vi "basic - VL Transmit.vi"() -> ()   [LabVIEW 2020]
uses:
  src/AIM664LV.lvlib
  src/_polimorphicInstances/session/Fdx Create Session (Tx-UDP Port-Oriented).vi
  src/bsp/AFDX_Transmit/Fdx Create Tx VL.vi
  src/_polimorphicInstances/udpPort/Fdx Create UDP Port (TX-CommPort).vi
  src/_polimorphicInstances/session/Fdx Close Session (Port).vi
  src/_controls/comm_computedMAC-IP.ctl
  src/_controls/comm_udp_tx.ctl
  src/_controls/comm_config_vl_tx.ctl
  src/helpers/EthFrameManagement/controls/mac_src_info_afdx.ctl
  src/helpers/EthFrameManagement/EthFrameManagement.lvlib
panel:
  in  "VlTx (IP Source)":T1={"domainID"=14, "sideID"=2, "locationID"=3, "interfaceID"=0}
  out "Duplicated":bool=TRUE
  in  "VL Configurations":T4(array[cluster])=[{"VL Config"={"VlId"=3, "NumOfSubVl"=2, "rate mS (128)"=128.0, "domainID"=1, "sideID"=1, "locationID"=254, "interfaceID"=1, "NetSelect"=3, "Skew"=0, "MaxFrameLength"=1000, "FrameBufferSize"=0}, "CommPort Config"=[{"PortType"=enum."FDX_UDP_SAMPLING", "partitionID"=0, "SubVlId"=1, "UdpSrcPort"=0, "UdpDstPort"=0, "SampleRateMs"=128.0, "UdpNumBufMessages"=0, "UdpMaxMessageSize"=1000}, {"PortType"=enum."FDX_UDP_SAMPLING", "partitionID"=0, "SubVlId"=2, "UdpSrcPort"=0, "UdpDstPort"=0, "SampleRateMs"=128.0, "UdpNumBufMessages"=0, "UdpMaxMessageSize"=1000}]}, {"VL Config"={"VlId"=70, "NumOfSubVl"=2, "rate mS (128)"=64.0, "domainID"=1, "sideID"=1, "locationID"=1, "interfaceID"=1, "NetSelect"=3, "Skew"=0, "MaxFrameLength"=1000, "FrameBufferSize"=0}, "CommPort Config"=[{"PortType"=enum."FDX_UDP_SAMPLING", "partitionID"=0, "SubVlId"=1, "UdpSrcPort"=0, "UdpDstPort"=0, "SampleRateMs"=128.0, "UdpNumBufMessages"=0, "UdpMaxMessageSize"=1000}, {"PortType"=enum."FDX_UDP_SAMPLING", "partitionID"=0, "SubVlId"=2, "UdpSrcPort"=0, "UdpDstPort"=0, "SampleRateMs"=128.0, "UdpNumBufMessages"=0, "UdpMaxMessageSize"=1000}]}] {"VL Config"."NetSelect" items=["FDX_TX_FRAME_DLY_A"=0, "FDX_TX_FRAME_DLY_B"=1, "FDX_TX_FRAME_BOTH "=3, "FDX_TX_FRAME_ONLY_A"=4, "FDX_TX_FRAME_ONLY_B "=5]; "VL Config"."interfaceID" format="%.0b"}
  in  "millisecond multiple":u32=128
  in  "PortMap":u32
  out "Data size":i32=128
  out "IndexCycleCount":u32[](array[numeric])
  out "MsgCount":u32[](array[numeric])=[13, 13, 21, 21]
  out "CurrentIndex":u32[](array[numeric])
  out "BytesWritten":u32[](array[numeric])=[128, 128, 128, 128]
  in  "Port":u32
  in  "Board":u32
  out "current time":timestamp=timestamp(3763148385.2241025 s since 1904-01-01)
  out "current irig time":T5={"SignOut"=-1509901600, "DayOut"=16, "HourOut"=8, "MinOut"=7, "SecondOut"=53, "MilliSecOut"=368, "MicroSecOut"=508, "NanoSecOut"=600, "InfoOut"=0, "Mode"=3}
  out "CommPort Addresses":T6[](array[typedef])=[{"MACsrc"=[], "IPsrc"="10.14.67.0", "IPdest"="224.224.0.3"}, {"MACsrc"=[], "IPsrc"="10.14.67.0", "IPdest"="224.224.0.3"}, {"MACsrc"=[], "IPsrc"="10.14.67.0", "IPdest"="224.224.0.70"}, {"MACsrc"=[], "IPsrc"="10.14.67.0", "IPdest"="224.224.0.70"}] {"MACsrc" format="%.0x"}
  out "Data":u8[](array[numeric])=[0, 1, 2, 3, 4, 5, 6, 7, 8, 9, 10, 11, 12, 13, 14, 15, 16, 17, 18, 19, 20, 21, 22, 23, 24, 25, 26, 27, 28, 29, 30, 31, 32, 33, 34, 35, 36, 37, 38, 39, 40, 41, 42, 43, 44, 45, 46, 47, 48, 49, 50, 51, 52, 53, 54, 55, 56, 57, 58, 59, 60, 61, 62, 63, 64, 65, 66, 67, 68, 69, 70, 71, 72, 73, 74, 75, 76, 77, 78, 79, 80, 81, 82, 83, 84, 85, 86, 87, 88, 89, 90, 91, 92, 93, 94, 95, 96, 97, 98, 99, 100, 101, 102, 103, 104, 105, 106, 107, 108, 109, 110, 111, 112, 113, 114, 115, 116, 117, 118, 119, 120, 121, 122, 123, 124, 125, 126, 127] format="%.0x"
  in  "stop":bool
  out "PortInitOut":T7={"PortConfig"=0, "PortUsed"=1, "GlobalMemFree"=0, "SharedMemFree"=0} {"PortConfig" items=["FDX_SINGLE", "FDX_REDUNDANT"]}
  out "error out":errorcluster
  # "ARINC 664 - Transmitting through many VL (Virtual Link)"
  # "Overview: Setup the board to transmit package as raw frames.\nRequirement: One AIM ARINC-664 board with installed AIM ARINC 664 BSP.\nRestrictions: None.\nInstruction:\n1. Select the Board ID (0 if you have only one board in your system) and the port number. If you want to validate between two ports in one device, you can use tx board and Rx Board\n2. Run the VI.\n3. See the result in Current IRIG Time"
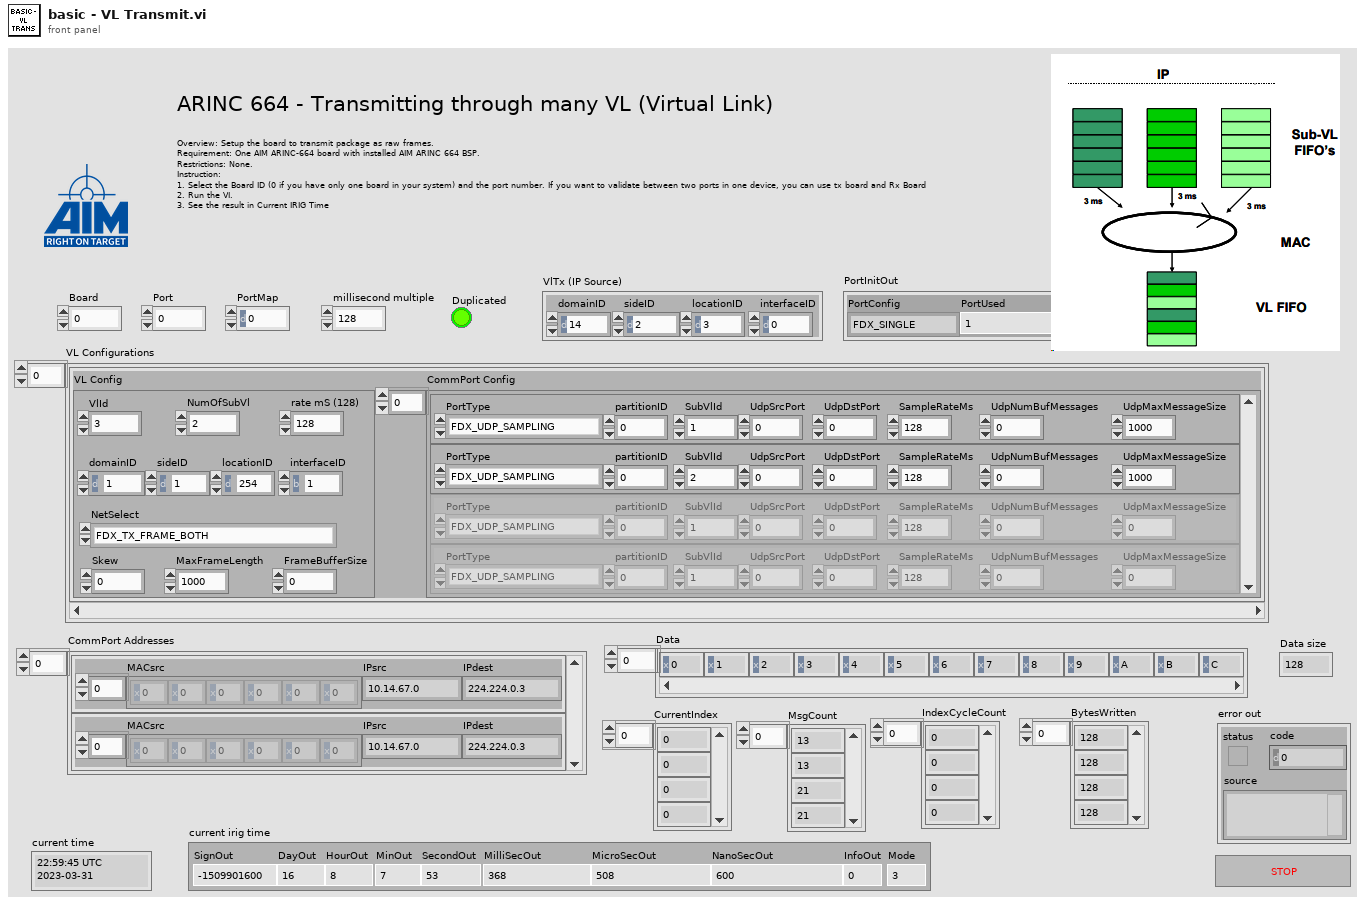
[diagram p1: front panel]
types:
  T1 = typedef "EthFrameManagement.lvlib/mac_src_info_afdx.ctl" = cluster{"domainID":u8, "sideID":u8, "locationID":u8, "interfaceID":u8}
  T2 = typedef "AIM664LV.lvlib/comm_config_vl_tx.ctl" = cluster{"VlId":u16, "NumOfSubVl":u16, "rate mS (128)":dbl, "domainID":u8, "sideID":u8, "locationID":u8, "interfaceID":u8, "NetSelect":u32, "Skew":u32, "MaxFrameLength":u32, "FrameBufferSize":u32}
  T3 = typedef "AIM664LV.lvlib/comm_udp_tx.ctl" = cluster{"PortType":enum16{"FDX_UDP_SAMPLING", "FDX_UDP_QUEUING"}, "partitionID":u8, "SubVlId":u8, "UdpSrcPort":u16, "UdpDstPort":u16, "SampleRateMs":dbl, "UdpNumBufMessages":u32, "UdpMaxMessageSize":u32}
  T4 = cluster{"VL Config":T2, "CommPort Config":T3[]}[]
  T5 = cluster{"SignOut":i32, "DayOut":u32, "HourOut":u32, "MinOut":u32, "SecondOut":u32, "MilliSecOut":u32, "MicroSecOut":u32, "NanoSecOut":u32, "InfoOut":u32, "Mode":u32}
  T6 = typedef "AIM664LV.lvlib/comm_computedMAC-IP.ctl" = cluster{"MACsrc":u8[], "IPsrc":string, "IPdest":string}
  T7 = cluster{"PortConfig":u32, "PortUsed":u32, "GlobalMemFree":u32, "SharedMemFree":u32}
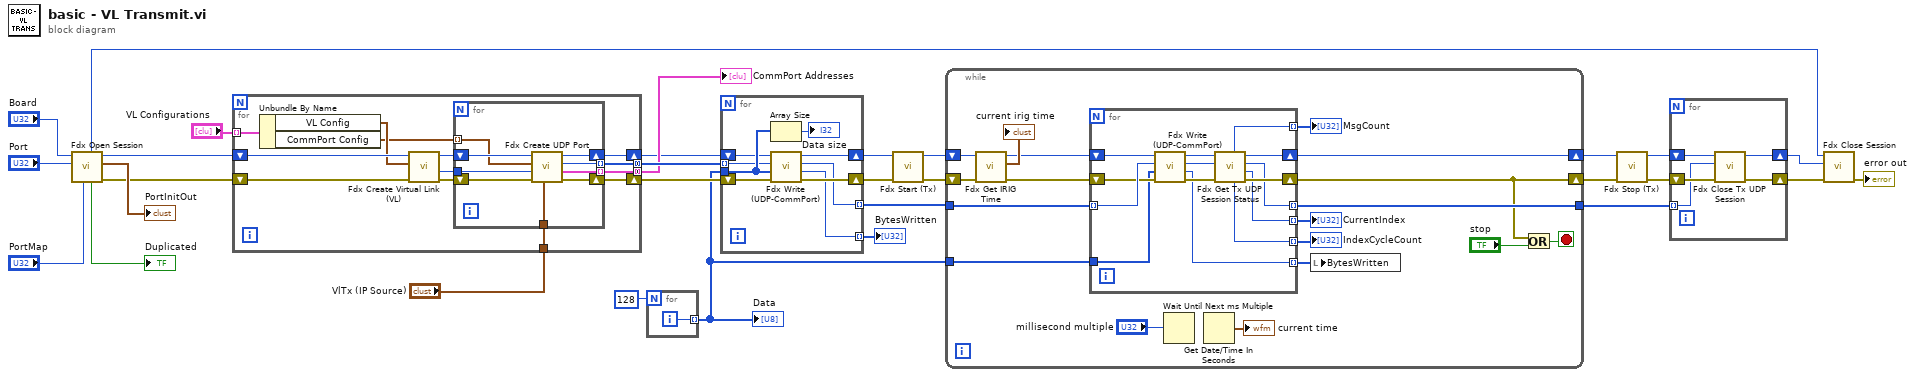
[diagram p0: block diagram]
diagram:
  n1 = call-poly "Fdx Open Session.vi"("PortMap"="PortMap", "port"="Port", "board"="Board") -> ("error out"=w12:errorcluster, "PortInitOut"=→"PortInitOut":T7, "port handle out"=w13:u32, "Duplicated"=→"Duplicated":bool, "InstrumentHandle_board out"=w5:u32)  [unwired: 4 in]
  n2 = for {
    tunnel: [w43] -> w28 mode=concatenating
    tunnel: [w41] -> w25 mode=concatenating
    tunnel: "VL Configurations" -> [w34] mode=indexing
    shift-right: [w35] -> w9
    shift-left: w13 -> [w40]
    shift-right: [w42] -> w26
    shift-left: w12 -> [w39]
    tunnel: "VlTx (IP Source)" -> [w31]
    n3 = Unbundle By Name(w34) -> ("VL Config"=w33:T2, "CommPort Config"=w32:T3[])
    n4 = call-poly "Fdx Create Virtual Link (VL).vi"("error in (no error)"=w39, "VL Config"=w33, "InstrumentHandle in"=w40) -> ("error out"=w37:errorcluster, "VlId"=w36:u16, "InstrumentHandle out"=w38:u32)  [unwired: 6 in]
    n5 = for {
      tunnel: [w51] -> w43 mode=indexing
      tunnel: [w48] -> w41 mode=indexing
      shift-right: [w47] -> w35
      shift-left: w38 -> [w52]
      shift-right: [w50] -> w42
      shift-left: w37 -> [w49]
      tunnel: w36 -> [w46]
      tunnel: w32 -> [w45] mode=indexing
      tunnel: w31 -> [w44]
      n6 = call-poly "Fdx Create UDP Port.vi"("VlTx"=w44, "error in (no error)"=w49, "VlId"=w46, "CommPort Config"=w45, "port handle in"=w52) -> ("error out"=w50:errorcluster, "computedAddresses"=w48:T6, "commPort handle out"=w51:u32, "port handle out"=w47:u32)  [unwired: 3 in]
    }
  }
  "CommPort Addresses" <- w25
  n7 = for {
    N: 128 -> [_]
    tunnel: [w53] -> w1 mode=indexing
    i -> [w53]
  }
  "Data" <- w1
  n8 = for {
    tunnel: w1 -> [w58]
    tunnel: [w60] -> w15 mode=indexing
    shift-right: [w61] -> w23
    shift-left: w26 -> [w62]
    tunnel: w28 -> [w57] mode=indexing
    tunnel: [w55] -> w27 mode=indexing
    shift-right: [w54] -> w4
    shift-left: w9 -> [w56]
    n9 = Array Size(array=w58) -> (size(s)=→"Data size":i32)
    n10 = call "Fdx Write (UDP-CommPort).vi"("error in (no error)"=w62, "Data"=w58, "UdpHandle in"=w57, "InstrumentHandle_port in"=w56) -> ("error out"=w61:errorcluster, "BytesWritten"=w60:u32, "UdpHandle out"=w55:u32, "InstrumentHandle_port out"=w54:u32)  [unwired: 4 in]
  }
  "BytesWritten" <- w15
  n11 = call "Fdx Start (Tx).vi"("error in (no error)"=w23, "InstrumentHandle_port in"=w4) -> ("error out"=w22:errorcluster, "InstrumentHandle_port out"=w21:u32)  [unwired: 8 in]
  n12 = while {
    tunnel: w27 -> [w68]
    tunnel: [w73] -> w18
    shift-right: [w64] -> w24
    shift-left: w21 -> [w77]
    shift-right: [w72] -> w19
    shift-left: w22 -> [w76]
    tunnel: w1 -> [w63]
    stop <- w79 stop-if-true
    n13 = call "Fdx Get IRIG Time.vi"("error in (no error)"=w76, "InstrumentHandle_board in"=w77) -> ("error out"=w67:errorcluster, "Curent Irig Time"=→"current irig time":T5, "InstrumentHandle_board out"=w65:u32)  [unwired: 7 in]
    n14 = for {
      tunnel: [w83] -> w73 mode=indexing
      tunnel: [w82] -> w71 mode=indexing
      tunnel: [w84] -> w70 mode=indexing
      tunnel: [w81] -> w69 mode=indexing
      tunnel: w68 -> [w93] mode=indexing
      tunnel: [w88] -> w66 mode=indexing
      tunnel: w63 -> [w90]
      shift-right: [w94] -> w72
      shift-left: w67 -> [w92]
      shift-right: [w85] -> w64
      shift-left: w65 -> [w89]
      n15 = call "Fdx Write (UDP-CommPort).vi"("error in (no error)"=w92, "Data"=w90, "UdpHandle in"=w93, "InstrumentHandle_port in"=w89) -> ("error out"=w91:errorcluster, "BytesWritten"=w88:u32, "UdpHandle out"=w87:u32, "InstrumentHandle_port out"=w86:u32)  [unwired: 4 in]
      n16 = call "Fdx Get Tx UDP Session Status.vi"("error in (no error)"=w91, "UdpHandle in"=w87, "InstrumentHandle_port in"=w86) -> ("error out"=w94:errorcluster, "CurrentIndex"=w82:u32, "UdpHandle out"=w83:u32, "InstrumentHandle_port out"=w85:u32, "IndexCycleCount"=w81:u32, "MsgCount"=w84:u32)  [unwired: 3 in]
    }
    "CurrentIndex" <- w71
    "MsgCount" <- w70
    "IndexCycleCount" <- w69
    n17 = Wait Until Next ms Multiple(millisecond multiple="millisecond multiple") -> ()  [unwired: 1 out]
    n18 = Get Date/Time In Seconds() -> (seconds since 1Jan1904=→"current time":timestamp)
    n19 = local write "BytesWritten"(w66) -> ()
    n20 = Or(x=w72, y="stop") -> (x .or. y?=w79:bool)
  }
  n21 = call "Fdx Stop (Tx).vi"("error in (no error)"=w19, "InstrumentHandle_port in"=w24) -> ("error out"=w17:errorcluster, "InstrumentHandle_port out"=w8:u32)  [unwired: 8 in]
  n22 = for {
    tunnel: w18 -> [w97] mode=indexing
    shift-right: [w98] -> w16
    shift-left: w17 -> [w99]
    shift-right: [w95] -> w7
    shift-left: w8 -> [w96]
    n23 = call "Fdx Close Tx UDP Session.vi"("error in (no error)"=w99, "UdpHandle in"=w97, "InstrumentHandle_port in"=w96) -> ("error out"=w98:errorcluster, "InstrumentHandle_port out"=w95:u32)  [unwired: 7 in]
  }
  n24 = call-poly "Fdx Close Session.vi"("error in (no error)"=w16, "InstrumentHandle_port in"=w7, "InstrumentHandle_board in"=w5) -> ("error out"=→"error out":errorcluster)  [unwired: 8 in]
